vi "Generate Simulated Data.vi"(8 "error in (no error)":errorcluster, 11 "Signal Type":T1) -> (0 "error out":errorcluster, 2 "Graph Data":waveform(dbl)[](array[waveform]))   [LabVIEW 2017, in "Acquisition.lvlib"]
doc: "Generates sample waveforms according to the signal type in the HW Config input."
uses:
  Acquisition.lvlib
  Signal Type.ctl
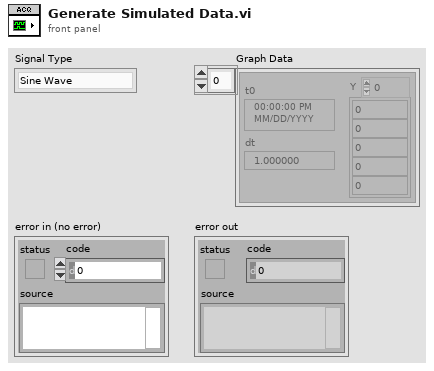
[diagram p1: front panel]
types:
  T1 = typedef "Acquisition.lvlib/Signal Type.ctl" = enum16{"Sine Wave", "Square with Noise"}
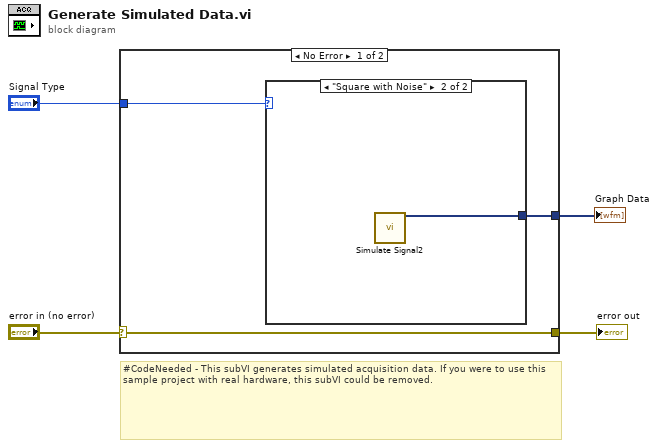
[diagram p0: block diagram]
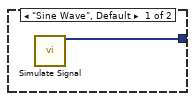
[diagram p2: hidden frame]
diagram:
  # "#CodeNeeded - This subVI generates simulated acquisition data. If you were to use this sample project with real hardware, this subVI could be removed."
  n1 = case shown="No Error" "error in (no error)" {
    selector: "error in (no error)" -> [w7 w10]
    tunnel: [w7 w10] -> w3
    tunnel: [w6 _] -> w2
    tunnel: "Signal Type" -> [w5 _]
    frame No Error {
      n2 = case shown="\"Square with Noise\"" w5 {
        tunnel: [w8 w9] -> w6
        frame "Sine Wave", Default {
          n3 = call "Simulate Signal"() -> ("Sine"=w8:dynamicdata)  [unwired: 14 in, 1 out]
        }
        frame "Square with Noise" {
          n4 = call "Simulate Signal2"() -> ("Square with Gaussian Noise"=w9:dynamicdata)  [unwired: 14 in, 1 out]
        }
      }
    }
    frame Error {
    }
  }
  "error out" <- w3
  "Graph Data" <- w2
